vi "Update data from CAN to CANFD.vi"(11 "CAN data":T1) -> (2 "Reset Command":bool, 3 "CAN_FD data":T2)   [LabVIEW 2025]
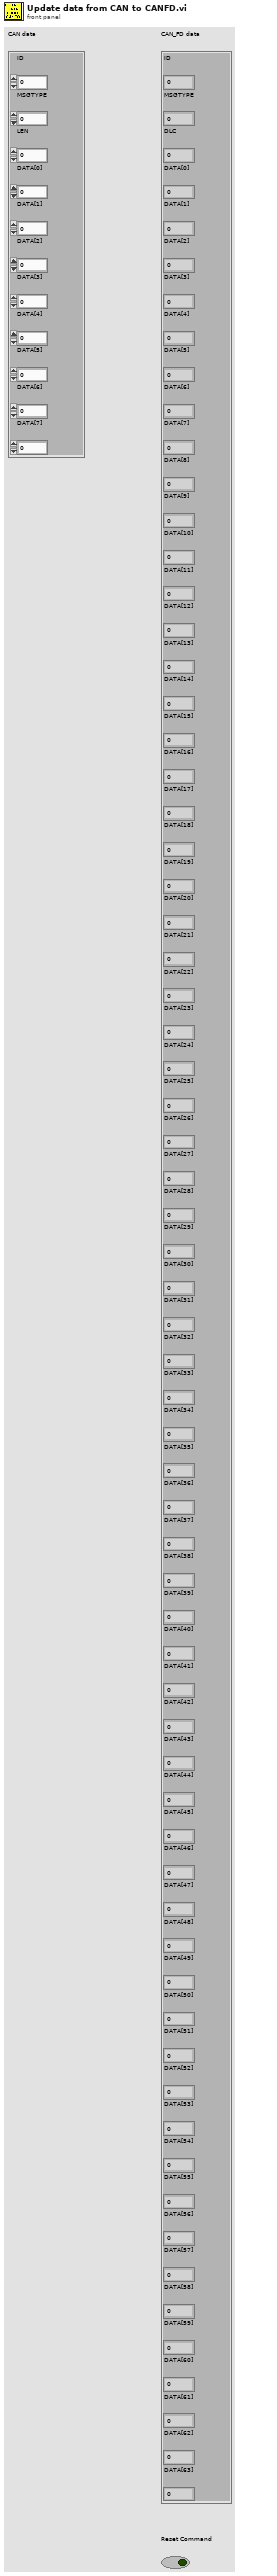
[diagram p1: front panel]
types:
  T1 = cluster{"ID":u32, "MSGTYPE":u8, "LEN":u8, "DATA[0]":u8, "DATA[1]":u8, "DATA[2]":u8, "DATA[3]":u8, "DATA[4]":u8, "DATA[5]":u8, "DATA[6]":u8, "DATA[7]":u8}
  T2 = cluster{"ID":u32, "MSGTYPE":u8, "DLC":u8, "DATA[0]":u8, "DATA[1]":u8, "DATA[2]":u8, "DATA[3]":u8, "DATA[4]":u8, "DATA[5]":u8, "DATA[6]":u8, "DATA[7]":u8, "DATA[8]":u8, "DATA[9]":u8, "DATA[10]":u8, "DATA[11]":u8, "DATA[12]":u8, "DATA[13]":u8, "DATA[14]":u8, "DATA[15]":u8, "DATA[16]":u8, "DATA[17]":u8, "DATA[18]":u8, "DATA[19]":u8, "DATA[20]":u8, "DATA[21]":u8, "DATA[22]":u8, "DATA[23]":u8, "DATA[24]":u8, "DATA[25]":u8, "DATA[26]":u8, "DATA[27]":u8, "DATA[28]":u8, "DATA[29]":u8, "DATA[30]":u8, "DATA[31]":u8, "DATA[32]":u8, "DATA[33]":u8, "DATA[34]":u8, "DATA[35]":u8, "DATA[36]":u8, "DATA[37]":u8, "DATA[38]":u8, "DATA[39]":u8, "DATA[40]":u8, "DATA[41]":u8, "DATA[42]":u8, "DATA[43]":u8, "DATA[44]":u8, "DATA[45]":u8, "DATA[46]":u8, "DATA[47]":u8, "DATA[48]":u8, "DATA[49]":u8, "DATA[50]":u8, "DATA[51]":u8, "DATA[52]":u8, "DATA[53]":u8, "DATA[54]":u8, "DATA[55]":u8, "DATA[56]":u8, "DATA[57]":u8, "DATA[58]":u8, "DATA[59]":u8, "DATA[60]":u8, "DATA[61]":u8, "DATA[62]":u8, "DATA[63]":u8}
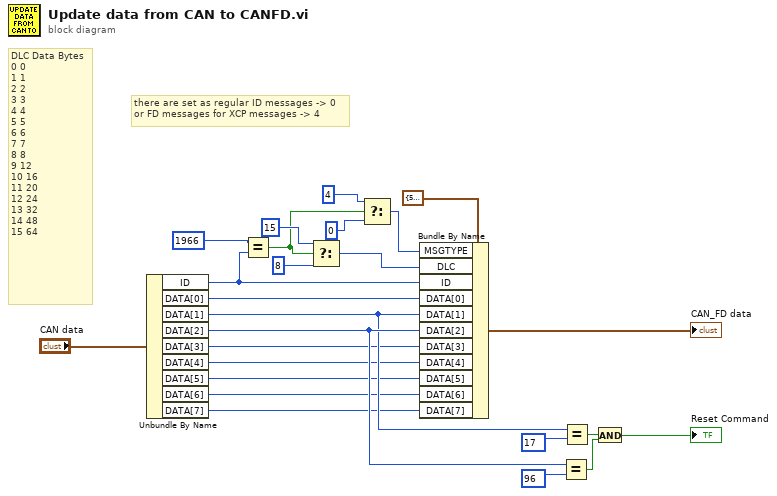
[diagram p0: block diagram]
diagram:
  # "DLC\tData Bytes\n0\t0\n1\t1\n2\t2\n3\t3\n4\t4\n5\t5\n6\t6\n7\t7\n8\t8\n9\t12\n10\t16\n11\t20\n12\t24\n13\t32\n14\t48\n15\t64"
  # "there are set as regular ID messages -> 0 \nor FD messages for XCP messages -> 4"
  n1 = Unbundle By Name("CAN data") -> ("ID"=w9:u32, "DATA[0]"=w11:u8, "DATA[1]"=w19:u8, "DATA[2]"=w20:u8, "DATA[3]"=w12:u8, "DATA[4]"=w13:u8, "DATA[5]"=w14:u8, "DATA[6]"=w15:u8, "DATA[7]"=w16:u8)
  n2 = Equal?(x=u32 1966, y=w9) -> (x = y?=w4:bool)
  n3 = Select(t=u8 15, s=w4, f=u8 8 ("DLC")) -> (s? t:f=w5:u8)
  n4 = Select(t=u8 4 ("MSGTYPE"), s=w4, f=u8 0 ("MSGTYPE")) -> (s? t:f=w1:u8)
  n5 = Bundle By Name(cluster=T2 {"ID"=507002890, "MSGTYPE"=2, "DLC"=0, "DATA[0]"=0, "DATA[1]"=0, "DATA[2]"=0, "DATA[3]"=0, "DATA[4]"=0, "DATA[5]"=0, "DATA[6]"=0, "DATA[7]"=0, "DATA[8]"=0, "DATA[9]"=0, "DATA[10]"=0, "DATA[11]"=0, "DATA[12]"=0, "DATA[13]"=0, "DATA[14]"=0, "DATA[15]"=0, "DATA[16]"=0, "DATA[17]"=0, "DATA[18]"=0, "DATA[19]"=0, "DATA[20]"=0, "DATA[21]"=0, "DATA[22]"=0, "DATA[23]"=0, "DATA[24]"=0, "DATA[25]"=0, "DATA[26]"=0, "DATA[27]"=0, "DATA[28]"=0, "DATA[29]"=0, "DATA[30]"=0, "DATA[31]"=0, "DATA[32]"=0, "DATA[33]"=0, "DATA[34]"=0, "DATA[35]"=0, "DATA[36]"=0, "DATA[37]"=0, "DATA[38]"=0, "DATA[39]"=0, "DATA[40]"=0, "DATA[41]"=0, "DATA[42]"=0, "DATA[43]"=0, "DATA[44]"=0, "DATA[45]"=0, "DATA[46]"=0, "DATA[47]"=0, "DATA[48]"=0, "DATA[49]"=0, "DATA[50]"=0, "DATA[51]"=0, "DATA[52]"=0, "DATA[53]"=0, "DATA[54]"=0, "DATA[55]"=0, "DATA[56]"=0, "DATA[57]"=0, "DATA[58]"=0, "DATA[59]"=0, "DATA[60]"=0, "DATA[61]"=0, "DATA[62]"=0, "DATA[63]"=0} ("MessageBuffer"), "MSGTYPE"=w1, "DLC"=w5, "ID"=w9, "DATA[0]"=w11, "DATA[1]"=w19, "DATA[2]"=w20, "DATA[3]"=w12, "DATA[4]"=w13, "DATA[5]"=w14, "DATA[6]"=w15, "DATA[7]"=w16) -> (→"CAN_FD data":T2)
  n6 = Equal?(x=w20, y=u8 96) -> (x = y?=w24:bool)
  n7 = Equal?(x=w19, y=u8 17) -> (x = y?=w23:bool)
  n8 = And(x=w23, y=w24) -> (x .and. y?=→"Reset Command":bool)
